vi "serviceMode_disable.vi"(8 "error in (no error)":errorcluster, 11 "Thorlabs_OSA200_64 in":refnum<class "OSA200.lvclass">) -> (0 "error out":errorcluster, 3 "Thorlabs_OSA200_64 out":refnum<class "OSA200.lvclass">)   [LabVIEW 2010, in "OSA200.lvclass"]
uses:
  OSA200.lvclass
  OSA.lvclass
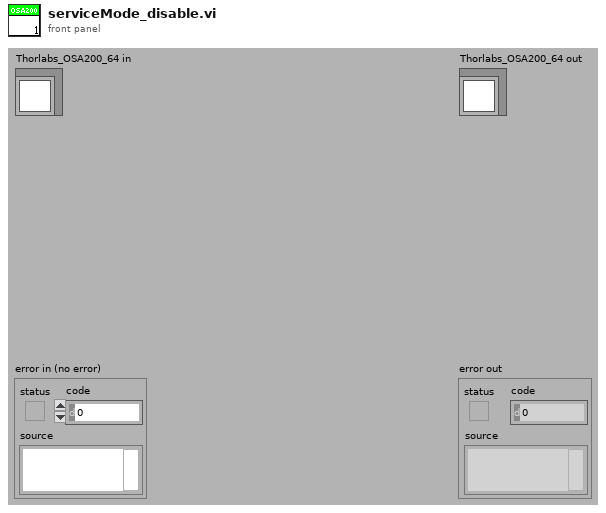
[diagram p1: front panel]
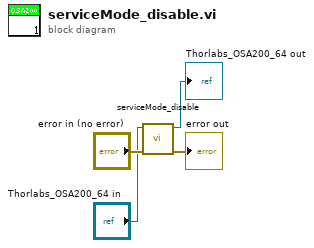
[diagram p0: block diagram]
diagram:
  n1 = call-parent "serviceMode_disable.vi"("error in (no error)"="error in (no error)", "Thorlabs_OSA_64 in"="Thorlabs_OSA200_64 in") -> ("error out"=→"error out":errorcluster, "Thorlabs_OSA_64 out"=→"Thorlabs_OSA200_64 out":refnum<class "OSA200.lvclass">)  [unwired: 8 in]
